vi "main.vi"() -> ()   [LabVIEW 2023]
doc: "This VI is a very simplistic example of how to use the KVaser CAN VIs. It uses all the required VIs to initialize the KVaser CAN library, open a CAN channel and configure the channel for use. The configuration of the channel is triggered by the user pressing the \"Go Bus On\" button. \n\nAt this point two different tasks are started. The first is task transmits the specified message when the \"Send Message\" button is pressed. The second task displays the last ten messages read on the channel. It is important to note that the messages transmitted by this channel will not show up in the received list.\n\nTo reconfigure the channel, \"Go Bus Off\", change the settings, and then \"Go Bus On\".\n\nTo stop execution, press \"Go Bus Off\". When the Bus Status LED is no longer lit, press the \"STOP\" button on the panel. This ensures that the hardware interface is freed correctly for the next application to use."
uses:
  readSub.ctl
panel:
  out "canArrayID_Out":string[](array[string])
  out "canArrayDataOut":string[](array[string])
  in  "Tab Control":enum32{"Page 1", "Page 2", "Page 3"}(tab)
  in  "Stop":bool
  in  "Data Bytes":u8[][](array[numeric])
  in  "Data Phase Bit Rate":i32(ring) items=["Classic 1M", "Classic 500K", "Classic 250K", "Classic 125K", "Classic 100K", "Classic 62K", "Classic 50K", "Classic 83K", "FD 500K", "FD 1M", "FD 2M", "FD 4M", "FD 8M"]
  in  "Arbitration Bit Rate":i32(ring) items=["Classic 1M", "Classic 500K", "Classic 250K", "Classic 125K", "Classic 100K", "Classic 62K", "Classic 50K", "Classic 83K", "FD 500K", "FD 1M", "FD 2M", "FD 4M", "FD 8M"]
  in  "Single Shot":bool
  in  "Bit Rate Switch":bool
  in  "FD Frame":bool
  in  "CAN FD NONISO":bool
  in  "CAN FD":bool
  in  "Accept Large DLC":bool
  in  "Wakeup":bool
  out "Read Error":errorcluster
  out "String":string
  in  "sendMessage":bool
  in  "Error Frame":bool
  in  "Extended Id":bool
  in  "Standard Id":bool
  in  "Remote Frame":bool
  out "Write Error":errorcluster
  in  "DLC":u8 max=64
  in  "Message Id":u32 max=536870911 format="%.0x"
  out "Bus Status":bool
  in  "Desired Bus State":bool
  in  "Channel #":bool caption="0"
  in  "Virtual":bool
  in  "Extended":bool
  in  "Exclusive":bool
  in  "flagCluster":T1
  in  "String 2":string="         2  1FFFFFFF   00000004    8        00\t00\tFF\tFF\tFF\tFF\tFF\tFF\r\n         3  0CF101A7   00000004    8        68\t00\t97\tCC\t00\t15\t39\t1A\r\n         2  1FFFFFFF   00000004    8        00\t00\tFF\tFF\tFF\tFF\tFF\tFF\r\n         3  0CF102A7   00000004    8        30\t75\tE0\t2E\t80\tFF\tFF\tFD\r\n         3  0CF101A7   00000004    8        68\t00\t97\tCC\t00\t15\t39\t1A\r\n         2  1FFFFFFF   00000004    8        00\t00\tFF\tFF\tFF\tFF\tFF\tFF\r\n        12  1FFFFFFF   00000004    8        00\t20\tFF\tFF\tFF\tFF\tFF\tFF\r\n         3  0CF102A7   00000004    8        30\t75\tE0\t2E\t80\tFF\tFF\tFD\r\n         3  0CF101A7   00000004    8        68\t00\t97\tCC\t00\t15\t39\t1A\r\n         2  1FFFFFFF   00000004    8        00\t00\tFF\tFF\tFF\tFF\tFF\tFF\r\n        22  1FFFFFFF   00000004    8        00\t20\tFF\tFF\tFF\tFF\tFF\tFF\r\n        12  1FFFFFFF   00000004    8        00\t20\tFF\tFF\tFF\tFF\tFF\tFF\r\n         3  0CF102A7   00000004    8        30\t75\tE0\t2E\t80\tFF\tFF\tFD\r\n         3  0CF101A7   00000004    8        68\t00\t97\tCC\t00\t15\t39\t1A\r\n         2  1FFFFFFF   00000004    8        00\t00\tFF\tFF\tFF\tFF\tFF\tFF\r\n        23  0CF101A7   00000004    8        68\t00\t97\tCC\t00\t15\t39\t1B\r\n        22  1FFFFFFF   00000004    8        00\t20\tFF\tFF\tFF\tFF\tFF\tFF\r\n        12  1FFFFFFF   00000004    8        00\t20\tFF\tFF\tFF\tFF\tFF\tFF\r\n         3  0CF102A7   00000004    8        30\t75\tE0\t2E\t80\tFF\tFF\tFD\r\n         3  0CF101A7   00000004    8        68\t00\t97\tCC\t00\t15\t39\t1A\r\n         2  1FFFFFFF   00000004    8        00\t00\tFF\tFF\tFF\tFF\tFF\tFF\r\n        23  0CF102A7   00000004    8        30\t75\tE0\t2E\t80\tFF\tFF\tFD\r\n        23  0CF101A7   00000004    8        68\t00\t97\tCC\t00\t15\t39\t1B\r\n        22  1FFFFFFF   00000004    8        00\t20\tFF\tFF\tFF\tFF\tFF\tFF\r\n        12  1FFFFFFF   00000004    8        00\t20\tFF\tFF\tFF\tFF\tFF\tFF\r\n         3  0CF102A7   00000004    8        30\t75\tE0\t2E\t80\tFF\tFF\tFD\r\n         3  0CF101A7   00000004    8        68\t00\t97\tCC\t00\t15\t39\t1A\r\n         2  1FFFFFFF   00000004    8        00\t00\tFF\tFF\tFF\tFF\tFF\tFF\r\n        32  1FFFFFFF   00000004    8        00\t20\tFF\tFF\tFF\tFF\tFF\tFF\r\n        23  0CF102A7   00000004    8        30\t75\tE0\t2E\t80\tFF\tFF\tFD\r\n        23  0CF101A7   00000004    8        68\t00\t97\tCC\t00\t15\t39\t1B\r\n        22  1FFFFFFF   00000004    8        00\t20\tFF\tFF\tFF\tFF\tFF\tFF\r\n        12  1FFFFFFF   00000004    8        00\t20\tFF\tFF\tFF\tFF\tFF\tFF\r\n         3  0CF102A7   00000004    8        30\t75\tE0\t2E\t80\tFF\tFF\tFD\r\n         3  0CF101A7   00000004    8        68\t00\t97\tCC\t00\t15\t39\t1A\r\n         2  1FFFFFFF   00000004    8        00\t00\tFF\tFF\tFF\tFF\tFF\tFF\r\n        41  18F11FF0   00000004    8        FF\t3F\t90\t68\t88\t1B\t10\t8C\r\n        32  1FFFFFFF   00000004    8        00\t20\tFF\tFF\tFF\tFF\tFF\tFF\r\n        23  0CF102A7   00000004    8        30\t75\tE0\t2E\t80\tFF\tFF\tFD\r\n        23  0CF101A7   00000004    8        68\t00\t97\tCC\t00\t15\t39\t1B\r\n        22  1FFFFFFF   00000004    8        00\t20\tFF\tFF\tFF\tFF\tFF\tFF\r\n        12  1FFFFFFF   00000004    8        00\t20\tFF\tFF\tFF\tFF\tFF\tFF\r\n         3  0CF102A7   00000004    8        30\t75\tE0\t2E\t80\tFF\tFF\tFD\r\n         3  0CF101A7   00000004    8        68\t00\t97\tCC\t00\t15\t39\t1A\r\n         2  1FFFFFFF   00000004    8        00\t00\tFF\tFF\tFF\tFF\tFF\tFF\r\n        42  18F120F0   00000004    8        2B\t75\t60\tB1\tB0\t01\tFF\tFF\r\n        41  18F11FF0   00000004    8        FF\t3F\t90\t68\t88\t1B\t10\t8C\r\n        32  1FFFFFFF   00000004    8        00\t20\tFF\tFF\tFF\tFF\tFF\tFF\r\n        23  0CF102A7   00000004    8        30\t75\tE0\t2E\t80\tFF\tFF\tFD\r\n        23  0CF101A7   00000004    8        68\t00\t97\tCC\t00\t15\t39\t1B\r\n        22  1FFFFFFF   00000004    8        00\t20\tFF\tFF\tFF\tFF\tFF\tFF\r\n        12  1FFFFFFF   00000004    8        00\t20\tFF\tFF\tFF\tFF\tFF\tFF\r\n         3  0CF102A7   00000004    8        30\t75\tE0\t2E\t80\tFF\tFF\tFD\r\n         3  0CF101A7   00000004    8        68\t00\t97\tCC\t00\t15\t39\t1A\r\n         2  1FFFFFFF   00000004    8        00\t00\tFF\tFF\tFF\tFF\tFF\tFF\r\n        43  0CF101A7   00000004    8        68\t00\t97\tCC\t00\t15\t39\t1C\r\n        42  18F120F0   00000004    8        2B\t75\t60\tB1\tB0\t01\tFF\tFF\r\n        41  18F11FF0   00000004    8        FF\t3F\t90\t68\t88\t1B\t10\t8C\r\n        32  1FFFFFFF   00000004    8        00\t20\tFF\tFF\tFF\tFF\tFF\tFF\r\n        23  0CF102A7   00000004    8        30\t75\tE0\t2E\t80\tFF\tFF\tFD\r\n        23  0CF101A7   00000004    8        68\t00\t97\tCC\t00\t15\t39\t1B\r\n        22  1FFFFFFF   00000004    8        00\t20\tFF\tFF\tFF\tFF\tFF\tFF\r\n        12  1FFFFFFF   00000004    8        00\t20\tFF\tFF\tFF\tFF\tFF\tFF\r\n         3  0CF102A7   00000004    8        30\t75\tE0\t2E\t80\tFF\tFF\tFD\r\n         3  0CF101A7   00000004    8        68\t00\t97\tCC\t00\t15\t39\t1A\r\n         2  1FFFFFFF   00000004    8        00\t00\tFF\tFF\tFF\tFF\tFF\tFF\r\n        43  0C3C4D4A   00000004    8        BE\tFF\tFF\t7F\t18\tFF\tFF\t38\r\n        43  0CF101A7   00000004    8        68\t00\t97\tCC\t00\t15\t39\t1C\r\n        42  18F120F0   00000004    8        2B\t75\t60\tB1\tB0\t01\tFF\tFF\r\n        41  18F11FF0   00000004    8        FF\t3F\t90\t68\t88\t1B\t10\t8C\r\n        32  1FFFFFFF   00000004    8        00\t20\tFF\tFF\tFF\tFF\tFF\tFF\r\n        23  0CF102A7   00000004    8        30\t75\tE0\t2E\t80\tFF\tFF\tFD\r\n        23  0CF101A7   00000004    8        68\t00\t97\tCC\t00\t15\t39\t1B\r\n        22  1FFFFFFF   00000004    8        00\t20\tFF\tFF\tFF\tFF\tFF\tFF\r\n        12  1FFFFFFF   00000004    8        00\t20\tFF\tFF\tFF\tFF\tFF\tFF\r\n         3  0CF102A7   00000004    8        30\t75\tE0\t2E\t80\tFF\tFF\tFD\r\n         3  0CF101A7   00000004    8        68\t00\t97\tCC\t00\t15\t39\t1A\r\n        44  0CF102A7   00000004    8        30\t75\tE0\t2E\t80\tFF\tFF\tFD\r\n        43  0C3C4D4A   00000004    8        BE\tFF\tFF\t7F\t18\tFF\tFF\t38\r\n        43  0CF101A7   00000004    8        68\t00\t97\tCC\t00\t15\t39\t1C\r\n        42  18F120F0   00000004    8        2B\t75\t60\tB1\tB0\t01\tFF\tFF\r\n        41  18F11FF0   00000004    8        FF\t3F\t90\t68\t88\t1B\t10\t8C\r\n        32  1FFFFFFF   00000004    8        00\t20\tFF\tFF\tFF\tFF\tFF\tFF\r\n        23  0CF102A7   00000004    8        30\t75\tE0\t2E\t80\tFF\tFF\tFD\r\n        23  0CF101A7   00000004    8        68\t00\t97\tCC\t00\t15\t39\t1B\r\n        22  1FFFFFFF   00000004    8        00\t20\tFF\tFF\tFF\tFF\tFF\tFF\r\n        12  1FFFFFFF   00000004    8        00\t20\tFF\tFF\tFF\tFF\tFF\tFF\r\n         3  0CF102A7   00000004    8        30\t75\tE0\t2E\t80\tFF\tFF\tFD\r\n        44  0CF103A7   00000004    8        17\t1F\t08\t60\tB1\t1F\t08\t38\r\n        44  0CF102A7   00000004    8        30\t75\tE0\t2E\t80\tFF\tFF\tFD\r\n        43  0C3C4D4A   00000004    8        BE\tFF\tFF\t7F\t18\tFF\tFF\t38\r\n        43  0CF101A7   00000004    8        68\t00\t97\tCC\t00\t15\t39\t1C\r\n        42  18F120F0   00000004    8        2B\t75\t60\tB1\tB0\t01\tFF\tFF\r\n        41  18F11FF0   00000004    8        FF\t3F\t90\t68\t88\t1B\t10\t8C\r\n        32  1FFFFFFF   00000004    8        00\t20\tFF\tFF\tFF\tFF\tFF\tFF\r\n        23  0CF102A7   00000004    8        30\t75\tE0\t2E\t80\tFF\tFF\tFD\r\n        23  0CF101A7   00000004    8        68\t00\t97\tCC\t00\t15\t39\t1B\r\n        22  1FFFFFFF   00000004    8        00\t20\tFF\tFF\tFF\tFF\tFF\tFF\r\n        12  1FFFFFFF   00000004    8        00\t20\tFF\tFF\tFF\tFF\tFF\tFF\r\n        45  0CF104A7   00000004    8        F0\t60\t22\tFC\tFF\tFF\tFF\t38\r\n        44  0CF103A7   00000004    8        17\t1F\t08\t60\tB1\t1F\t08\t38\r\n        44  0CF102A7   00000004    8        30\t75\tE0\t2E\t80\tFF\tFF\tFD\r\n        43  0C3C4D4A   00000004    8        BE\tFF\tFF\t7F\t18\tFF\tFF\t38\r\n        43  0CF101A7   00000004    8        68\t00\t97\tCC\t00\t15\t39\t1C\r\n        42  18F120F0   00000004    8        2B\t75\t60\tB1\tB0\t01\tFF\tFF\r\n        41  18F11FF0   00000004    8        FF\t3F\t90\t68\t88\t1B\t10\t8C\r\n        32  1FFFFFFF   00000004    8        00\t20\tFF\tFF\tFF\tFF\tFF\tFF\r\n        23  0CF102A7   00000004    8        30\t75\tE0\t2E\t80\tFF\tFF\tFD\r\n        23  0CF101A7   00000004    8        68\t00\t97\tCC\t00\t15\t39\t1B\r\n        22  1FFFFFFF   00000004    8        00\t20\tFF\tFF\tFF\tFF\tFF\tFF\r\n        46  18F106A7   00000004    8        00\tF7\tFF\tFF\tFF\tFF\tFF\t71\r\n        45  0CF104A7   00000004    8        F0\t60\t22\tFC\tFF\tFF\tFF\t38\r\n        44  0CF103A7   00000004    8        17\t1F\t08\t60\tB1\t1F\t08\t38\r\n        44  0CF102A7   00000004    8        30\t75\tE0\t2E\t80\tFF\tFF\tFD\r\n        43  0C3C4D4A   00000004    8        BE\tFF\tFF\t7F\t18\tFF\tFF\t38\r\n        43  0CF101A7   00000004    8        68\t00\t97\tCC\t00\t15\t39\t1C\r\n        42  18F120F0   00000004    8        2B\t75\t60\tB1\tB0\t01\tFF\tFF\r\n        41  18F11FF0   00000004    8        FF\t3F\t90\t68\t88\t1B\t10\t8C\r\n        32  1FFFFFFF   00000004    8        00\t20\tFF\tFF\tFF\tFF\tFF\tFF\r\n        23  0CF102A7   00000004    8        30\t75\tE0\t2E\t80\tFF\tFF\tFD\r\n        23  0CF101A7   00000004    8        68\t00\t97\tCC\t00\t15\t39\t1B\r\n        46  18F121F0   00000004    8        09\t16\t00\t00\tFF\tFF\tB0\t01\r\n        46  18F106A7   00000004    8        00\tF7\tFF\tFF\tFF\tFF\tFF\t71\r\n        45  0CF104A7   00000004    8        F0\t60\t22\tFC\tFF\tFF\tFF\t38\r\n        44  0CF103A7   00000004    8        17\t1F\t08\t60\tB1\t1F\t08\t38\r\n        44  0CF102A7   00000004    8        30\t75\tE0\t2E\t80\tFF\tFF\tFD\r\n        43  0C3C4D4A   00000004    8        BE\tFF\tFF\t7F\t18\tFF\tFF\t38\r\n        43  0CF101A7   00000004    8        68\t00\t97\tCC\t00\t15\t39\t1C\r\n        42  18F120F0   00000004    8        2B\t75\t60\tB1\tB0\t01\tFF\tFF\r\n        41  18F11FF0   00000004    8        FF\t3F\t90\t68\t88\t1B\t10\t8C\r\n        32  1FFFFFFF   00000004    8        00\t20\tFF\tFF\tFF\tFF\tFF\tFF\r\n        23  0CF102A7   00000004    8        30\t75\tE0\t2E\t80\tFF\tFF\tFD\r\n        47  1FFFFFFF   00000004    8        00\t00\tFF\tFF\tFF\tFF\tFF\tFF\r\n        46  18F121F0   00000004    8        09\t16\t00\t00\tFF\tFF\tB0\t01\r\n        46  18F106A7   00000004    8        00\tF7\tFF\tFF\tFF\tFF\tFF\t71\r\n        45  0CF104A7   00000004    8        F0\t60\t22\tFC\tFF\tFF\tFF\t38\r\n        44  0CF103A7   00000004    8        17\t1F\t08\t60\tB1\t1F\t08\t38\r\n        44  0CF102A7   00000004    8        30\t75\tE0\t2E\t80\tFF\tFF\tFD\r\n        43  0C3C4D4A   00000004    8        BE\tFF\tFF\t7F\t18\tFF\tFF\t38\r\n        43  0CF101A7   00000004    8        68\t00\t97\tCC\t00\t15\t39\t1C\r\n        42  18F120F0   00000004    8        2B\t75\t60\tB1\tB0\t01\tFF\tFF\r\n        41  18F11FF0   00000004    8        FF\t3F\t90\t68\t88\t1B\t10\t8C\r\n        32  1FFFFFFF   00000004    8        00\t20\tFF\tFF\tFF\tFF\tFF\tFF\r\n        52  1FFFFFFF   00000004    8        00\t00\tFF\tFF\tFF\tFF\tFF\tFF\r\n        47  1FFFFFFF   00000004    8        00\t00\tFF\tFF\tFF\tFF\tFF\tFF\r\n        46  18F121F0   00000004    8        09\t16\t00\t00\tFF\tFF\tB0\t01\r\n        46  18F106A7   00000004    8        00\tF7\tFF\tFF\tFF\tFF\tFF\t71\r\n        45  0CF104A7   00000004    8        F0\t60\t22\tFC\tFF\tFF\tFF\t38\r\n        44  0CF103A7   00000004    8        17\t1F\t08\t60\tB1\t1F\t08\t38\r\n        44  0CF102A7   00000004    8        30\t75\tE0\t2E\t80\tFF\tFF\tFD\r\n        43  0C3C4D4A   00000004    8        BE\tFF\tFF\t7F\t18\tFF\tFF\t38\r\n        43  0CF101A7   00000004    8        68\t00\t97\tCC\t00\t15\t39\t1C\r\n        42  18F120F0   00000004    8        2B\t75\t60\tB1\tB0\t01\tFF\tFF\r\n        41  18F11FF0   00000004    8        FF\t3F\t90\t68\t88\t1B\t10\t8C\r\n        62  1FFFFFFF   00000004    8        00\t20\tFF\tFF\tFF\tFF\tFF\tFF\r\n        52  1FFFFFFF   00000004    8        00\t00\tFF\tFF\tFF\tFF\tFF\tFF\r\n        47  1FFFFFFF   00000004    8        00\t00\tFF\tFF\tFF\tFF\tFF\tFF\r\n        46  18F121F0   00000004    8        09\t16\t00\t00\tFF\tFF\tB0\t01\r\n        46  18F106A7   00000004    8        00\tF7\tFF\tFF\tFF\tFF\tFF\t71\r\n        45  0CF104A7   00000004    8        F0\t60\t22\tFC\tFF\tFF\tFF\t38\r\n        44  0CF103A7   00000004    8        17\t1F\t08\t60\tB1\t1F\t08\t38\r\n        44  0CF102A7   00000004    8        30\t75\tE0\t2E\t80\tFF\tFF\tFD\r\n        43  0C3C4D4A   00000004    8        BE\tFF\tFF\t7F\t18\tFF\tFF\t38\r\n        43  0CF101A7   00000004    8        68\t00\t97\tCC\t00\t15\t39\t1C\r\n        42  18F120F0   00000004    8        2B\t75\t60\tB1\tB0\t01\tFF\tFF\r\n        63  0CF101A7   00000004    8        68\t00\t97\tCC\t00\t15\t39\t1D\r\n        62  1FFFFFFF   00000004    8        00\t20\tFF\tFF\tFF\tFF\tFF\tFF\r\n        52  1FFFFFFF   00000004    8        00\t00\tFF\tFF\tFF\tFF\tFF\tFF\r\n        47  1FFFFFFF   00000004    8        00\t00\tFF\tFF\tFF\tFF\tFF\tFF\r\n        46  18F121F0   00000004    8        09\t16\t00\t00\tFF\tFF\tB0\t01\r\n        46  18F106A7   00000004    8        00\tF7\tFF\tFF\tFF\tFF\tFF\t71\r\n        45  0CF104A7   00000004    8        F0\t60\t22\tFC\tFF\tFF\tFF\t38\r\n        44  0CF103A7   00000004    8        17\t1F\t08\t60\tB1\t1F\t08\t38\r\n        44  0CF102A7   00000004    8        30\t75\tE0\t2E\t80\tFF\tFF\tFD\r\n        43  0C3C4D4A   00000004    8        BE\tFF\tFF\t7F\t18\tFF\tFF\t38\r\n        43  0CF101A7   00000004    8        68\t00\t97\tCC\t00\t15\t39\t1C\r\n        63  0CF102A7   00000004    8        30\t75\tE0\t2E\t80\tFF\tFF\tFD\r\n        63  0CF101A7   00000004    8        68\t00\t97\tCC\t00\t15\t39\t1D\r\n        62  1FFFFFFF   00000004    8        00\t20\tFF\tFF\tFF\tFF\tFF\tFF\r\n        52  1FFFFFFF   00000004    8        00\t00\tFF\tFF\tFF\tFF\tFF\tFF\r\n        47  1FFFFFFF   00000004    8        00\t00\tFF\tFF\tFF\tFF\tFF\tFF\r\n        46  18F121F0   00000004    8        09\t16\t00\t00\tFF\tFF\tB0\t01\r\n        46  18F106A7   00000004    8        00\tF7\tFF\tFF\tFF\tFF\tFF\t71\r\n        45  0CF104A7   00000004    8        F0\t60\t22\tFC\tFF\tFF\tFF\t38\r\n        44  0CF103A7   00000004    8        17\t1F\t08\t60\tB1\t1F\t08\t38\r\n        44  0CF102A7   00000004    8        30\t75\tE0\t2E\t80\tFF\tFF\tFD\r\n        43  0C3C4D4A   00000004    8        BE\tFF\tFF\t7F\t18\tFF\tFF\t38\r\n        72  1FFFFFFF   00000004    8        00\t00\tFF\tFF\tFF\tFF\tFF\tFF\r\n        63  0CF102A7   00000004    8        30\t75\tE0\t2E\t80\tFF\tFF\tFD\r\n        63  0CF101A7   00000004    8        68\t00\t97\tCC\t00\t15\t39\t1D\r\n        62  1FFFFFFF   00000004    8        00\t20\tFF\tFF\tFF\tFF\tFF\tFF\r\n        52  1FFFFFFF   00000004    8        00\t00\tFF\tFF\tFF\tFF\tFF\tFF\r\n        47  1FFFFFFF   00000004    8        00\t00\tFF\tFF\tFF\tFF\tFF\tFF\r\n        46  18F121F0   00000004    8        09\t16\t00\t00\tFF\tFF\tB0\t01\r\n        46  18F106A7   00000004    8        00\tF7\tFF\tFF\tFF\tFF\tFF\t71\r\n        45  0CF104A7   00000004    8        F0\t60\t22\tFC\tFF\tFF\tFF\t38\r\n        44  0CF103A7   00000004    8        17\t1F\t08\t60\tB1\t1F\t08\t38\r\n        44  0CF102A7   00000004    8        30\t75\tE0\t2E\t80\tFF\tFF\tFD\r\n        82  1FFFFFFF   00000004    8        00\t20\tFF\tFF\tFF\tFF\tFF\tFF\r\n        72  1FFFFFFF   00000004    8        00\t00\tFF\tFF\tFF\tFF\tFF\tFF\r\n        63  0CF102A7   00000004    8        30\t75\tE0\t2E\t80\tFF\tFF\tFD\r\n        63  0CF101A7   00000004    8        68\t00\t97\tCC\t00\t15\t39\t1D\r\n        62  1FFFFFFF   00000004    8        00\t20\tFF\tFF\tFF\tFF\tFF\tFF\r\n        52  1FFFFFFF   00000004    8        00\t00\tFF\tFF\tFF\tFF\tFF\tFF\r\n        47  1FFFFFFF   00000004    8        00\t00\tFF\tFF\tFF\tFF\tFF\tFF\r\n        46  18F121F0   00000004    8        09\t16\t00\t00\tFF\tFF\tB0\t01\r\n        46  18F106A7   00000004    8        00\tF7\tFF\tFF\tFF\tFF\tFF\t71\r\n        45  0CF104A7   00000004    8        F0\t60\t22\tFC\tFF\tFF\tFF\t38\r\n        44  0CF103A7   00000004    8        17\t1F\t08\t60\tB1\t1F\t08\t38\r\n        83  0CF101A7   00000004    8        68\t00\t97\tCC\t00\t15\t39\t1E\r\n        82  1FFFFFFF   00000004    8        00\t20\tFF\tFF\tFF\tFF\tFF\tFF\r\n        72  1FFFFFFF   00000004    8        00\t00\tFF\tFF\tFF\tFF\tFF\tFF\r\n        63  0CF102A7   00000004    8        30\t75\tE0\t2E\t80\tFF\tFF\tFD\r\n        63  0CF101A7   00000004    8        68\t00\t97\tCC\t00\t15\t39\t1D\r\n        62  1FFFFFFF   00000004    8        00\t20\tFF\tFF\tFF\tFF\tFF\tFF\r\n        52  1FFFFFFF   00000004    8        00\t00\tFF\tFF\tFF\tFF\tFF\tFF\r\n        47  1FFFFFFF   00000004    8        00\t00\tFF\tFF\tFF\tFF\tFF\tFF\r\n        46  18F121F0   00000004    8        09\t16\t00\t00\tFF\tFF\tB0\t01\r\n        46  18F106A7   00000004    8        00\tF7\tFF\tFF\tFF\tFF\tFF\t71\r\n        45  0CF104A7   00000004    8        F0\t60\t22\tFC\tFF\tFF\tFF\t38\r\n        83  0CF102A7   00000004    8        30\t75\tE0\t2E\t80\tFF\tFF\tFD\r\n        83  0CF101A7   00000004    8        68\t00\t97\tCC\t00\t15\t39\t1E\r\n        82  1FFFFFFF   00000004    8        00\t20\tFF\tFF\tFF\tFF\tFF\tFF\r\n        72  1FFFFFFF   00000004    8        00\t00\tFF\tFF\tFF\tFF\tFF\tFF\r\n        63  0CF102A7   00000004    8        30\t75\tE0\t2E\t80\tFF\tFF\tFD\r\n        63  0CF101A7   00000004    8        68\t00\t97\tCC\t00\t15\t39\t1D\r\n        62  1FFFFFFF   00000004    8        00\t20\tFF\tFF\tFF\tFF\tFF\tFF\r\n        52  1FFFFFFF   00000004    8        00\t00\tFF\tFF\tFF\tFF\tFF\tFF\r\n        47  1FFFFFFF   00000004    8        00\t00\tFF\tFF\tFF\tFF\tFF\tFF\r\n        46  18F121F0   00000004    8        09\t16\t00\t00\tFF\tFF\tB0\t01\r\n        46  18F106A7   00000004    8        00\tF7\tFF\tFF\tFF\tFF\tFF\t71\r\n        92  1FFFFFFF   00000004    8        00\t00\tFF\tFF\tFF\tFF\tFF\tFF\r\n        83  0CF102A7   00000004    8        30\t75\tE0\t2E\t80\tFF\tFF\tFD\r\n        83  0CF101A7   00000004    8        68\t00\t97\tCC\t00\t15\t39\t1E\r\n        82  1FFFFFFF   00000004    8        00\t20\tFF\tFF\tFF\tFF\tFF\tFF\r\n        72  1FFFFFFF   00000004    8        00\t00\tFF\tFF\tFF\tFF\tFF\tFF\r\n        63  0CF102A7   00000004    8        30\t75\tE0\t2E\t80\tFF\tFF\tFD\r\n        63  0CF101A7   00000004    8        68\t00\t97\tCC\t00\t15\t39\t1D\r\n        62  1FFFFFFF   00000004    8        00\t20\tFF\tFF\tFF\tFF\tFF\tFF\r\n        52  1FFFFFFF   00000004    8        00\t00\tFF\tFF\tFF\tFF\tFF\tFF\r\n        47  1FFFFFFF   00000004    8        00\t00\tFF\tFF\tFF\tFF\tFF\tFF\r\n        46  18F121F0   00000004    8        09\t16\t00\t00\tFF\tFF\tB0\t01\r\n        93  18F106A7   00000004    8        00\tF7\tFF\tFF\tFF\tFF\tFF\t72\r\n        92  1FFFFFFF   00000004    8        00\t00\tFF\tFF\tFF\tFF\tFF\tFF\r\n        83  0CF102A7   00000004    8        30\t75\tE0\t2E\t80\tFF\tFF\tFD\r\n        83  0CF101A7   00000004    8        68\t00\t97\tCC\t00\t15\t39\t1E\r\n        82  1FFFFFFF   00000004    8        00\t20\tFF\tFF\tFF\tFF\tFF\tFF\r\n        72  1FFFFFFF   00000004    8        00\t00\tFF\tFF\tFF\tFF\tFF\tFF\r\n        63  0CF102A7   00000004    8        30\t75\tE0\t2E\t80\tFF\tFF\tFD\r\n        63  0CF101A7   00000004    8        68\t00\t97\tCC\t00\t15\t39\t1D\r\n        62  1FFFFFFF   00000004    8        00\t20\tFF\tFF\tFF\tFF\tFF\tFF\r\n        52  1FFFFFFF   00000004    8        00\t00\tFF\tFF\tFF\tFF\tFF\tFF\r\n        47  1FFFFFFF   00000004    8        00\t00\tFF\tFF\tFF\tFF\tFF\tFF\r\n       102  1FFFFFFF   00000004    8        00\t20\tFF\tFF\tFF\tFF\tFF\tFF\r\n        93  18F106A7   00000004    8        00\tF7\tFF\tFF\tFF\tFF\tFF\t72\r\n        92  1FFFFFFF   00000004    8        00\t00\tFF\tFF\tFF\tFF\tFF\tFF\r\n        83  0CF102A7   00000004    8        30\t75\tE0\t2E\t80\tFF\tFF\tFD\r\n        83  0CF101A7   00000004    8        68\t00\t97\tCC\t00\t15\t39\t1E\r\n        82  1FFFFFFF   00000004    8        00\t20\tFF\tFF\tFF\tFF\tFF\tFF\r\n        72  1FFFFFFF   00000004    8        00\t00\tFF\tFF\tFF\tFF\tFF\tFF\r\n        63  0CF102A7   00000004    8        30\t75\tE0\t2E\t80\tFF\tFF\tFD\r\n        63  0CF101A7   00000004    8        68\t00\t97\tCC\t00\t15\t39\t1D\r\n        62  1FFFFFFF   00000004    8        00\t20\tFF\tFF\tFF\tFF\tFF\tFF\r\n        52  1FFFFFFF   00000004    8        00\t00\tFF\tFF\tFF\tFF\tFF\tFF\r\n       103  0CF101A7   00000004    8        68\t00\t97\tCC\t00\t15\t39\t1F\r\n       102  1FFFFFFF   00000004    8        00\t20\tFF\tFF\tFF\tFF\tFF\tFF\r\n        93  18F106A7   00000004    8        00\tF7\tFF\tFF\tFF\tFF\tFF\t72\r\n        92  1FFFFFFF   00000004    8        00\t00\tFF\tFF\tFF\tFF\tFF\tFF\r\n        83  0CF102A7   00000004    8        30\t75\tE0\t2E\t80\tFF\tFF\tFD\r\n        83  0CF101A7   00000004    8        68\t00\t97\tCC\t00\t15\t39\t1E\r\n        82  1FFFFFFF   00000004    8        00\t20\tFF\tFF\tFF\tFF\tFF\tFF\r\n        72  1FFFFFFF   00000004    8        00\t00\tFF\tFF\tFF\tFF\tFF\tFF\r\n        63  0CF102A7   00000004    8        30\t75\tE0\t2E\t80\tFF\tFF\tFD\r\n        63  0CF101A7   00000004    8        68\t00\t97\tCC\t00\t15\t39\t1D\r\n        62  1FFFFFFF   00000004    8        00\t20\tFF\tFF\tFF\tFF\tFF\tFF\r\n       103  0CF102A7   00000004    8        30\t75\tE0\t2E\t80\tFF\tFF\tFD\r\n       103  0CF101A7   00000004    8        68\t00\t97\tCC\t00\t15\t39\t1F\r\n       102  1FFFFFFF   00000004    8        00\t20\tFF\tFF\tFF\tFF\tFF\tFF\r\n        93  18F106A7   00000004    8        00\tF7\tFF\tFF\tFF\tFF\tFF\t72\r\n        92  1FFFFFFF   00000004    8        00\t00\tFF\tFF\tFF\tFF\tFF\tFF\r\n        83  0CF102A7   00000004    8        30\t75\tE0\t2E\t80\tFF\tFF\tFD\r\n        83  0CF101A7   00000004    8        68\t00\t97\tCC\t00\t15\t39\t1E\r\n        82  1FFFFFFF   00000004    8        00\t20\tFF\tFF\tFF\tFF\tFF\tFF\r\n        72  1FFFFFFF   00000004    8        00\t00\tFF\tFF\tFF\tFF\tFF\tFF\r\n        63  0CF102A7   00000004    8        30\t75\tE0\t2E\t80\tFF\tFF\tFD\r\n        63  0CF101A7   00000004    8        68\t00\t97\tCC\t00\t15\t39\t1D\r\n       112  1FFFFFFF   00000004    8        00\t20\tFF\tFF\tFF\tFF\tFF\tFF\r\n       103  0CF102A7   00000004    8        30\t75\tE0\t2E\t80\tFF\tFF\tFD\r\n       103  0CF101A7   00000004    8        68\t00\t97\tCC\t00\t15\t39\t1F\r\n       102  1FFFFFFF   00000004    8        00\t20\tFF\tFF\tFF\tFF\tFF\tFF\r\n        93  18F106A7   00000004    8        00\tF7\tFF\tFF\tFF\tFF\tFF\t72\r\n        92  1FFFFFFF   00000004    8        00\t00\tFF\tFF\tFF\tFF\tFF\tFF\r\n        83  0CF102A7   00000004    8        30\t75\tE0\t2E\t80\tFF\tFF\tFD\r\n        83  0CF101A7   00000004    8        68\t00\t97\tCC\t00\t15\t39\t1E\r\n        82  1FFFFFFF   00000004    8        00\t20\tFF\tFF\tFF\tFF\tFF\tFF\r\n        72  1FFFFFFF   00000004    8        00\t00\tFF\tFF\tFF\tFF\tFF\tFF\r\n        63  0CF102A7   00000004    8        30\t75\tE0\t2E\t80\tFF\tFF\tFD\r\n       122  1FFFFFFF   00000004    8        00\t00\tFF\tFF\tFF\tFF\tFF\tFF\r\n       112  1FFFFFFF   00000004    8        00\t20\tFF\tFF\tFF\tFF\tFF\tFF\r\n       103  0CF102A7   00000004    8        30\t75\tE0\t2E\t80\tFF\tFF\tFD\r\n       103  0CF101A7   00000004    8        68\t00\t97\tCC\t00\t15\t39\t1F\r\n       102  1FFFFFFF   00000004    8        00\t20\tFF\tFF\tFF\tFF\tFF\tFF\r\n        93  18F106A7   00000004    8        00\tF7\tFF\tFF\tFF\tFF\tFF\t72\r\n        92  1FFFFFFF   00000004    8        00\t00\tFF\tFF\tFF\tFF\tFF\tFF\r\n        83  0CF102A7   00000004    8        30\t75\tE0\t2E\t80\tFF\tFF\tFD\r\n        83  0CF101A7   00000004    8        68\t00\t97\tCC\t00\t15\t39\t1E\r\n        82  1FFFFFFF   00000004    8        00\t20\tFF\tFF\tFF\tFF\tFF\tFF\r\n        72  1FFFFFFF   00000004    8        00\t00\tFF\tFF\tFF\tFF\tFF\tFF\r\n       123  0CF101A7   00000004    8        68\t00\t97\tCC\t00\t15\t39\t20\r\n       122  1FFFFFFF   00000004    8        00\t00\tFF\tFF\tFF\tFF\tFF\tFF\r\n       112  1FFFFFFF   00000004    8        00\t20\tFF\tFF\tFF\tFF\tFF\tFF\r\n       103  0CF102A7   00000004    8        30\t75\tE0\t2E\t80\tFF\tFF\tFD\r\n       103  0CF101A7   00000004    8        68\t00\t97\tCC\t00\t15\t39\t1F\r\n       102  1FFFFFFF   00000004    8        00\t20\tFF\tFF\tFF\tFF\tFF\tFF\r\n        93  18F106A7   00000004    8        00\tF7\tFF\tFF\tFF\tFF\tFF\t72\r\n        92  1FFFFFFF   00000004    8        00\t00\tFF\tFF\tFF\tFF\tFF\tFF\r\n        83  0CF102A7   00000004    8        30\t75\tE0\t2E\t80\tFF\tFF\tFD\r\n        83  0CF101A7   00000004    8        68\t00\t97\tCC\t00\t15\t39\t1E\r\n        82  1FFFFFFF   00000004    8        00\t20\tFF\tFF\tFF\tFF\tFF\tFF\r\n       123  0CF102A7   00000004    8        30\t75\tE0\t2E\t80\tFF\tFF\tFD\r\n       123  0CF101A7   00000004    8        68\t00\t97\tCC\t00\t15\t39\t20\r\n       122  1FFFFFFF   00000004    8        00\t00\tFF\tFF\tFF\tFF\tFF\tFF\r\n       112  1FFFFFFF   00000004    8        00\t20\tFF\tFF\tFF\tFF\tFF\tFF\r\n       103  0CF102A7   00000004    8        30\t75\tE0\t2E\t80\tFF\tFF\tFD\r\n       103  0CF101A7   00000004    8        68\t00\t97\tCC\t00\t15\t39\t1F\r\n       102  1FFFFFFF   00000004    8        00\t20\tFF\tFF\tFF\tFF\tFF\tFF\r\n        93  18F106A7   00000004    8        00\tF7\tFF\tFF\tFF\tFF\tFF\t72\r\n        92  1FFFFFFF   00000004    8        00\t00\tFF\tFF\tFF\tFF\tFF\tFF\r\n        83  0CF102A7   00000004    8        30\t75\tE0\t2E\t80\tFF\tFF\tFD\r\n        83  0CF101A7   00000004    8        68\t00\t97\tCC\t00\t15\t39\t1E\r\n       132  1FFFFFFF   00000004    8        00\t20\tFF\tFF\tFF\tFF\tFF\tFF\r\n       123  0CF102A7   00000004    8        30\t75\tE0\t2E\t80\tFF\tFF\tFD\r\n       123  0CF101A7   00000004    8        68\t00\t97\tCC\t00\t15\t39\t20\r\n       122  1FFFFFFF   00000004    8        00\t00\tFF\tFF\tFF\tFF\tFF\tFF\r\n       112  1FFFFFFF   00000004    8        00\t20\tFF\tFF\tFF\tFF\tFF\tFF\r\n       103  0CF102A7   00000004    8        30\t75\tE0\t2E\t80\tFF\tFF\tFD\r\n       103  0CF101A7   00000004    8        68\t00\t97\tCC\t00\t15\t39\t1F\r\n       102  1FFFFFFF   00000004    8        00\t20\tFF\tFF\tFF\tFF\tFF\tFF\r\n        93  18F106A7   00000004    8        00\tF7\tFF\tFF\tFF\tFF\tFF\t72\r\n        92  1FFFFFFF   00000004    8        00\t00\tFF\tFF\tFF\tFF\tFF\tFF\r\n        83  0CF102A7   00000004    8        30\t75\tE0\t2E\t80\tFF\tFF\tFD\r\n       141  18F11FF0   00000004    8        FF\t3F\t90\t68\t88\t1B\t10\t9C\r\n       132  1FFFFFFF   00000004    8        00\t20\tFF\tFF\tFF\tFF\tFF\tFF\r\n       123  0CF102A7   00000004    8        30\t75\tE0\t2E\t80\tFF\tFF\tFD\r\n       123  0CF101A7   00000004    8        68\t00\t97\tCC\t00\t15\t39\t20\r\n       122  1FFFFFFF   00000004    8        00\t00\tFF\tFF\tFF\tFF\tFF\tFF\r\n       112  1FFFFFFF   00000004    8        00\t20\tFF\tFF\tFF\tFF\tFF\tFF\r\n       103  0CF102A7   00000004    8        30\t75\tE0\t2E\t80\tFF\tFF\tFD\r\n       103  0CF101A7   00000004    8        68\t00\t97\tCC\t00\t15\t39\t1F\r\n       102  1FFFFFFF   00000004    8        00\t20\tFF\tFF\tFF\tFF\tFF\tFF\r\n        93  18F106A7   00000004    8        00\tF7\tFF\tFF\tFF\tFF\tFF\t72\r\n        92  1FFFFFFF   00000004    8        00\t00\tFF\tFF\tFF\tFF\tFF\tFF\r\n       142  18F120F0   00000004    8        2B\t75\t60\tB1\tB0\t01\tFF\tFF\r\n       141  18F11FF0   00000004    8        FF\t3F\t90\t68\t88\t1B\t10\t9C\r\n       132  1FFFFFFF   00000004    8        00\t20\tFF\tFF\tFF\tFF\tFF\tFF\r\n       123  0CF102A7   00000004    8        30\t75\tE0\t2E\t80\tFF\tFF\tFD\r\n       123  0CF101A7   00000004    8        68\t00\t97\tCC\t00\t15\t39\t20\r\n       122  1FFFFFFF   00000004    8        00\t00\tFF\tFF\tFF\tFF\tFF\tFF\r\n       112  1FFFFFFF   00000004    8        00\t20\tFF\tFF\tFF\tFF\tFF\tFF\r\n       103  0CF102A7   00000004    8        30\t75\tE0\t2E\t80\tFF\tFF\tFD\r\n       103  0CF101A7   00000004    8        68\t00\t97\tCC\t00\t15\t39\t1F\r\n       102  1FFFFFFF   00000004    8        00\t20\tFF\tFF\tFF\tFF\tFF\tFF\r\n        93  18F106A7   00000004    8        00\tF7\tFF\tFF\tFF\tFF\tFF\t72\r\n       143  0CF101A7   00000004    8        68\t00\t97\tCC\t00\t15\t39\t21\r\n       142  18F120F0   00000004    8        2B\t75\t60\tB1\tB0\t01\tFF\tFF\r\n       141  18F11FF0   00000004    8        FF\t3F\t90\t68\t88\t1B\t10\t9C\r\n       132  1FFFFFFF   00000004    8        00\t20\tFF\tFF\tFF\tFF\tFF\tFF\r\n       123  0CF102A7   00000004    8        30\t75\tE0\t2E\t80\tFF\tFF\tFD\r\n       123  0CF101A7   00000004    8        68\t00\t97\tCC\t00\t15\t39\t20\r\n       122  1FFFFFFF   00000004    8        00\t00\tFF\tFF\tFF\tFF\tFF\tFF\r\n       112  1FFFFFFF   00000004    8        00\t20\tFF\tFF\tFF\tFF\tFF\tFF\r\n       103  0CF102A7   00000004    8        30\t75\tE0\t2E\t80\tFF\tFF\tFD\r\n       103  0CF101A7   00000004    8        68\t00\t97\tCC\t00\t15\t39\t1F\r\n       102  1FFFFFFF   00000004    8        00\t20\tFF\tFF\tFF\tFF\tFF\tFF\r\n       143  0C3C4D4A   00000004    8        BE\tFF\tFF\t7F\t18\tFF\tFF\t39\r\n       143  0CF101A7   00000004    8        68\t00\t97\tCC\t00\t15\t39\t21\r\n       142  18F120F0   00000004    8        2B\t75\t60\tB1\tB0\t01\tFF\tFF\r\n       141  18F11FF0   00000004    8        FF\t3F\t90\t68\t88\t1B\t10\t9C\r\n       132  1FFFFFFF   00000004    8        00\t20\tFF\tFF\tFF\tFF\tFF\tFF\r\n       123  0CF102A7   00000004    8        30\t75\tE0\t2E\t80\tFF\tFF\tFD\r\n       123  0CF101A7   00000004    8        68\t00\t97\tCC\t00\t15\t39\t20\r\n       122  1FFFFFFF   00000004    8        00\t00\tFF\tFF\tFF\tFF\tFF\tFF\r\n       112  1FFFFFFF   00000004    8        00\t20\tFF\tFF\tFF\tFF\tFF\tFF\r\n       103  0CF102A7   00000004    8        30\t75\tE0\t2E\t80\tFF\tFF\tFD\r\n       103  0CF101A7   00000004    8        68\t00\t97\tCC\t00\t15\t39\t1F\r\n       144  0CF102A7   00000004    8        30\t75\tE0\t2E\t80\tFF\tFF\tFD\r\n       143  0C3C4D4A   00000004    8        BE\tFF\tFF\t7F\t18\tFF\tFF\t39\r\n       143  0CF101A7   00000004    8        68\t00\t97\tCC\t00\t15\t39\t21\r\n       142  18F120F0   00000004    8        2B\t75\t60\tB1\tB0\t01\tFF\tFF\r\n       141  18F11FF0   00000004    8        FF\t3F\t90\t68\t88\t1B\t10\t9C\r\n       132  1FFFFFFF   00000004    8        00\t20\tFF\tFF\tFF\tFF\tFF\tFF\r\n       123  0CF102A7   00000004    8        30\t75\tE0\t2E\t80\tFF\tFF\tFD\r\n       123  0CF101A7   00000004    8        68\t00\t97\tCC\t00\t15\t39\t20\r\n       122  1FFFFFFF   00000004    8        00\t00\tFF\tFF\tFF\tFF\tFF\tFF\r\n       112  1FFFFFFF   00000004    8        00\t20\tFF\tFF\tFF\tFF\tFF\tFF\r\n       103  0CF102A7   00000004    8        30\t75\tE0\t2E\t80\tFF\tFF\tFD\r\n       144  0CF103A7   00000004    8        17\t1F\t08\t60\tB1\t1F\t08\t39\r\n       144  0CF102A7   00000004    8        30\t75\tE0\t2E\t80\tFF\tFF\tFD\r\n       143  0C3C4D4A   00000004    8        BE\tFF\tFF\t7F\t18\tFF\tFF\t39\r\n       143  0CF101A7   00000004    8        68\t00\t97\tCC\t00\t15\t39\t21\r\n       142  18F120F0   00000004    8        2B\t75\t60\tB1\tB0\t01\tFF\tFF\r\n       141  18F11FF0   00000004    8        FF\t3F\t90\t68\t88\t1B\t10\t9C\r\n       132  1FFFFFFF   00000004    8        00\t20\tFF\tFF\tFF\tFF\tFF\tFF\r\n       123  0CF102A7   00000004    8        30\t75\tE0\t2E\t80\tFF\tFF\tFD\r\n       123  0CF101A7   00000004    8        68\t00\t97\tCC\t00\t15\t39\t20\r\n       122  1FFFFFFF   00000004    8        00\t00\tFF\tFF\tFF\tFF\tFF\tFF\r\n       112  1FFFFFFF   00000004    8        00\t20\tFF\tFF\tFF\tFF\tFF\tFF\r\n       145  0CF104A7   00000004    8        F0\t60\t22\tFC\tFF\tFF\tFF\t39\r\n       144  0CF103A7   00000004    8        17\t1F\t08\t60\tB1\t1F\t08\t39\r\n       144  0CF102A7   00000004    8        30\t75\tE0\t2E\t80\tFF\tFF\tFD\r\n       143  0C3C4D4A   00000004    8        BE\tFF\tFF\t7F\t18\tFF\tFF\t39\r\n       143  0CF101A7   00000004    8        68\t00\t97\tCC\t00\t15\t39\t21\r\n       142  18F120F0   00000004    8        2B\t75\t60\tB1\tB0\t01\tFF\tFF\r\n       141  18F11FF0   00000004    8        FF\t3F\t90\t68\t88\t1B\t10\t9C\r\n       132  1FFFFFFF   00000004    8        00\t20\tFF\tFF\tFF\tFF\tFF\tFF\r\n       123  0CF102A7   00000004    8        30\t75\tE0\t2E\t80\tFF\tFF\tFD\r\n       123  0CF101A7   00000004    8        68\t00\t97\tCC\t00\t15\t39\t20\r\n       122  1FFFFFFF   00000004    8        00\t00\tFF\tFF\tFF\tFF\tFF\tFF\r\n       145  18F106A7   00000004    8        00\tF7\tFF\tFF\tFF\tFF\tFF\t73\r\n       145  0CF104A7   00000004    8        F0\t60\t22\tFC\tFF\tFF\tFF\t39\r\n       144  0CF103A7   00000004    8        17\t1F\t08\t60\tB1\t1F\t08\t39\r\n       144  0CF102A7   00000004    8        30\t75\tE0\t2E\t80\tFF\tFF\tFD\r\n       143  0C3C4D4A   00000004    8        BE\tFF\tFF\t7F\t18\tFF\tFF\t39\r\n       143  0CF101A7   00000004    8        68\t00\t97\tCC\t00\t15\t39\t21\r\n       142  18F120F0   00000004    8        2B\t75\t60\tB1\tB0\t01\tFF\tFF\r\n       141  18F11FF0   00000004    8        FF\t3F\t90\t68\t88\t1B\t10\t9C\r\n       132  1FFFFFFF   00000004    8        00\t20\tFF\tFF\tFF\tFF\tFF\tFF\r\n       123  0CF102A7   00000004    8        30\t75\tE0\t2E\t80\tFF\tFF\tFD\r\n       123  0CF101A7   00000004    8        68\t00\t97\tCC\t00\t15\t39\t20\r\n       146  18F108A7   00000004    8        F0\t00\t00\tFF\tFF\tFF\tFF\t3E\r\n       145  18F106A7   00000004    8        00\tF7\tFF\tFF\tFF\tFF\tFF\t73\r\n       145  0CF104A7   00000004    8        F0\t60\t22\tFC\tFF\tFF\tFF\t39\r\n       144  0CF103A7   00000004    8        17\t1F\t08\t60\tB1\t1F\t08\t39\r\n       144  0CF102A7   00000004    8        30\t75\tE0\t2E\t80\tFF\tFF\tFD\r\n       143  0C3C4D4A   00000004    8        BE\tFF\tFF\t7F\t18\tFF\tFF\t39\r\n       143  0CF101A7   00000004    8        68\t00\t97\tCC\t00\t15\t39\t21\r\n       142  18F120F0   00000004    8        2B\t75\t60\tB1\tB0\t01\tFF\tFF\r\n       141  18F11FF0   00000004    8        FF\t3F\t90\t68\t88\t1B\t10\t9C\r\n       132  1FFFFFFF   00000004    8        00\t20\tFF\tFF\tFF\tFF\tFF\tFF\r\n       123  0CF102A7   00000004    8        30\t75\tE0\t2E\t80\tFF\tFF\tFD\r\n       147  18F121F0   00000004    8        09\t16\t00\t00\tFF\tFF\tB0\t01\r\n       146  18F108A7   00000004    8        F0\t00\t00\tFF\tFF\tFF\tFF\t3E\r\n       145  18F106A7   00000004    8        00\tF7\tFF\tFF\tFF\tFF\tFF\t73\r\n       145  0CF104A7   00000004    8        F0\t60\t22\tFC\tFF\tFF\tFF\t39\r\n       144  0CF103A7   00000004    8        17\t1F\t08\t60\tB1\t1F\t08\t39\r\n       144  0CF102A7   00000004    8        30\t75\tE0\t2E\t80\tFF\tFF\tFD\r\n       143  0C3C4D4A   00000004    8        BE\tFF\tFF\t7F\t18\tFF\tFF\t39\r\n       143  0CF101A7   00000004    8        68\t00\t97\tCC\t00\t15\t39\t21\r\n       142  18F120F0   00000004    8        2B\t75\t60\tB1\tB0\t01\tFF\tFF\r\n       141  18F11FF0   00000004    8        FF\t3F\t90\t68\t88\t1B\t10\t9C\r\n       132  1FFFFFFF   00000004    8        00\t20\tFF\tFF\tFF\tFF\tFF\tFF\r\n       147  18FEF117   00000004    8        F7\t97\tCC\tCF\tFF\tFF\tFF\tFF\r\n       147  18F121F0   00000004    8        09\t16\t00\t00\tFF\tFF\tB0\t01\r\n       146  18F108A7   00000004    8        F0\t00\t00\tFF\tFF\tFF\tFF\t3E\r\n       145  18F106A7   00000004    8        00\tF7\tFF\tFF\tFF\tFF\tFF\t73\r\n       145  0CF104A7   00000004    8        F0\t60\t22\tFC\tFF\tFF\tFF\t39\r\n       144  0CF103A7   00000004    8        17\t1F\t08\t60\tB1\t1F\t08\t39\r\n       144  0CF102A7   00000004    8        30\t75\tE0\t2E\t80\tFF\tFF\tFD\r\n       143  0C3C4D4A   00000004    8        BE\tFF\tFF\t7F\t18\tFF\tFF\t39\r\n       143  0CF101A7   00000004    8        68\t00\t97\tCC\t00\t15\t39\t21\r\n       142  18F120F0   00000004    8        2B\t75\t60\tB1\tB0\t01\tFF\tFF\r\n       141  18F11FF0   00000004    8        FF\t3F\t90\t68\t88\t1B\t10\t9C\r\n       148  1FFFFFFF   00000004    8        00\t00\tFF\tFF\tFF\tFF\tFF\tFF\r\n       147  18FEF117   00000004    8        F7\t97\tCC\tCF\tFF\tFF\tFF\tFF\r\n       147  18F121F0   00000004    8        09\t16\t00\t00\tFF\tFF\tB0\t01\r\n       146  18F108A7   00000004    8        F0\t00\t00\tFF\tFF\tFF\tFF\t3E\r\n       145  18F106A7   00000004    8        00\tF7\tFF\tFF\tFF\tFF\tFF\t73\r\n       145  0CF104A7   00000004    8        F0\t60\t22\tFC\tFF\tFF\tFF\t39\r\n       144  0CF103A7   00000004    8        17\t1F\t08\t60\tB1\t1F\t08\t39\r\n       144  0CF102A7   00000004    8        30\t75\tE0\t2E\t80\tFF\tFF\tFD\r\n       143  0C3C4D4A   00000004    8        BE\tFF\tFF\t7F\t18\tFF\tFF\t39\r\n       143  0CF101A7   00000004    8        68\t00\t97\tCC\t00\t15\t39\t21\r\n       142  18F120F0   00000004    8        2B\t75\t60\tB1\tB0\t01\tFF\tFF\r\n       152  1FFFFFFF   00000004    8        00\t20\tFF\tFF\tFF\tFF\tFF\tFF\r\n       148  1FFFFFFF   00000004    8        00\t00\tFF\tFF\tFF\tFF\tFF\tFF\r\n       147  18FEF117   00000004    8        F7\t97\tCC\tCF\tFF\tFF\tFF\tFF\r\n       147  18F121F0   00000004    8        09\t16\t00\t00\tFF\tFF\tB0\t01\r\n       146  18F108A7   00000004    8        F0\t00\t00\tFF\tFF\tFF\tFF\t3E\r\n       145  18F106A7   00000004    8        00\tF7\tFF\tFF\tFF\tFF\tFF\t73\r\n       145  0CF104A7   00000004    8        F0\t60\t22\tFC\tFF\tFF\tFF\t39\r\n       144  0CF103A7   00000004    8        17\t1F\t08\t60\tB1\t1F\t08\t39\r\n       144  0CF102A7   00000004    8        30\t75\tE0\t2E\t80\tFF\tFF\tFD\r\n       143  0C3C4D4A   00000004    8        BE\tFF\tFF\t7F\t18\tFF\tFF\t39\r\n       143  0CF101A7   00000004    8        68\t00\t97\tCC\t00\t15\t39\t21\r\n       162  1FFFFFFF   00000004    8        00\t00\tFF\tFF\tFF\tFF\tFF\tFF\r\n       152  1FFFFFFF   00000004    8        00\t20\tFF\tFF\tFF\tFF\tFF\tFF\r\n       148  1FFFFFFF   00000004    8        00\t00\tFF\tFF\tFF\tFF\tFF\tFF\r\n       147  18FEF117   00000004    8        F7\t97\tCC\tCF\tFF\tFF\tFF\tFF\r\n       147  18F121F0   00000004    8        09\t16\t00\t00\tFF\tFF\tB0\t01\r\n       146  18F108A7   00000004    8        F0\t00\t00\tFF\tFF\tFF\tFF\t3E\r\n       145  18F106A7   00000004    8        00\tF7\tFF\tFF\tFF\tFF\tFF\t73\r\n       145  0CF104A7   00000004    8        F0\t60\t22\tFC\tFF\tFF\tFF\t39\r\n       144  0CF103A7   00000004    8        17\t1F\t08\t60\tB1\t1F\t08\t39\r\n       144  0CF102A7   00000004    8        30\t75\tE0\t2E\t80\tFF\tFF\tFD\r\n       143  0C3C4D4A   00000004    8        BE\tFF\tFF\t7F\t18\tFF\tFF\t39\r\n       163  0CF101A7   00000004    8        68\t00\t97\tCC\t00\t15\t39\t22\r\n       162  1FFFFFFF   00000004    8        00\t00\tFF\tFF\tFF\tFF\tFF\tFF\r\n       152  1FFFFFFF   00000004    8        00\t20\tFF\tFF\tFF\tFF\tFF\tFF\r\n       148  1FFFFFFF   00000004    8        00\t00\tFF\tFF\tFF\tFF\tFF\tFF\r\n       147  18FEF117   00000004    8        F7\t97\tCC\tCF\tFF\tFF\tFF\tFF\r\n       147  18F121F0   00000004    8        09\t16\t00\t00\tFF\tFF\tB0\t01\r\n       146  18F108A7   00000004    8        F0\t00\t00\tFF\tFF\tFF\tFF\t3E\r\n       145  18F106A7   00000004    8        00\tF7\tFF\tFF\tFF\tFF\tFF\t73\r\n       145  0CF104A7   00000004    8        F0\t60\t22\tFC\tFF\tFF\tFF\t39\r\n       144  0CF103A7   00000004    8        17\t1F\t08\t60\tB1\t1F\t08\t39\r\n       144  0CF102A7   00000004    8        30\t75\tE0\t2E\t80\tFF\tFF\tFD\r\n       163  0CF102A7   00000004    8        30\t75\tE0\t2E\t80\tFF\tFF\tFD\r\n       163  0CF101A7   00000004    8        68\t00\t97\tCC\t00\t15\t39\t22\r\n       162  1FFFFFFF   00000004    8        00\t00\tFF\tFF\tFF\tFF\tFF\tFF\r\n       152  1FFFFFFF   00000004    8        00\t20\tFF\tFF\tFF\tFF\tFF\tFF\r\n       148  1FFFFFFF   00000004    8        00\t00\tFF\tFF\tFF\tFF\tFF\tFF\r\n       147  18FEF117   00000004    8        F7\t97\tCC\tCF\tFF\tFF\tFF\tFF\r\n       147  18F121F0   00000004    8   
